vi "PSLDAQ_Close.vi"(0 "Handle In":T1) -> ()   [LabVIEW 2010]
doc: "1. 설명\n a. 장치와 통신 연결 기능 비활성화 및 할당된 메모리 제거\n\n2. 기능\n a. PSLDAQ_Open 함수에서 할당된 메모리, 쓰레드 제거\n b. PSL-DAQ 장치와 통신 연결 비활성화, 모든 기능 중지\n \n3. 터미널\n a. 터미널 입력\n ○ Handle In : 장치 핸들\n\n4. 주의\n a. PSLDAQ_Open 함수를 사용한 경우 반드시 PSLDAQ_Close 함수를 사용해야 함. \n b. 모든 함수를 사용한 후 호출함.\n c. PSLDAQ_Close 함수 사용 후 다시 PSLDAQ_Open 함수 사용 가능"
uses:
  PSLDAQ_Dll.dll
panel:
  # "PSLDAQ_Close\n\n1. 설명\n  a. 장치와 통신 연결 기능 비활성화 및 할당된 메모리 제거\n\n2. 기능\n  a. PSLDAQ_Open 함수에서 할당된 메모리, 쓰레드 제거\n  b. PSL-DAQ 장치와 통신 연결 비활성화, 모든 기능 중지\n        \n3. 터미널\n  a. 터미널 입력\n    ○ Handle In : 장치 핸들\n\n4. 주의\n  a. PSLDAQ_Open 함수를 사용한 경우 반드시 PSLDAQ_Close 함수를 사용해야 함.  \n  b. 모든 함수를 사용한 후 호출함.\n  c. PSLDAQ_Close 함수 사용 후 다시 PSLDAQ_Open 함수 사용 가능"
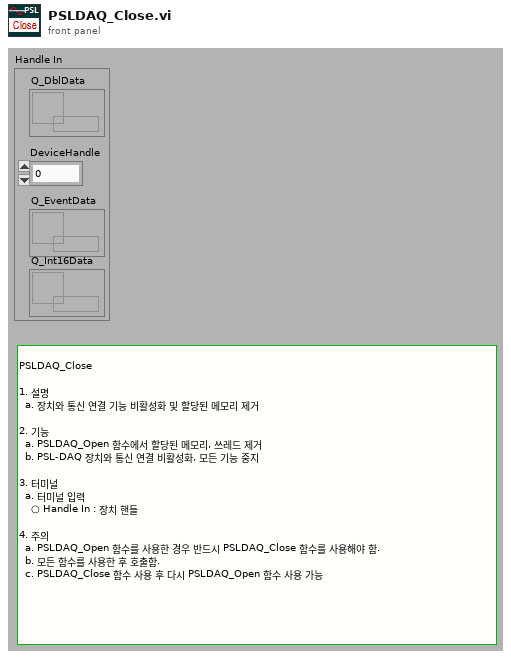
[diagram p1: front panel]
types:
  T1 = cluster{"Q_DblData":refnum<queue>, "DeviceHandle":u32, "Q_EventData":refnum<queue>, "Q_Int16Data":refnum<queue>}
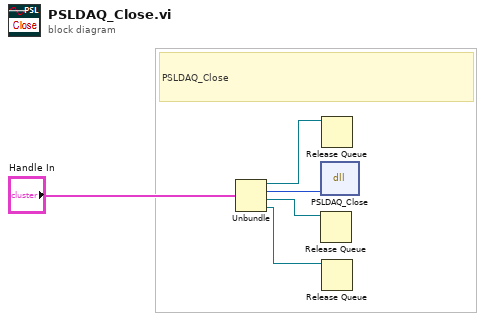
[diagram p0: block diagram]
diagram:
  # "PSLDAQ_Close"
  n1 = Unbundle("Handle In") -> ("Q_DblData"=w3:refnum<queue>, "DeviceHandle"=w5:u32, "Q_EventData"=w4:refnum<queue>, "Q_Int16Data"=w1:refnum<queue>)
  n2 = dll-call lib="D:/PSL-DAQ LabVIEW Library/PSLDAQ_Dll.dll" fn="PSLDAQ_Close"("DeviceHandle"=w5) -> ()  [unwired: 5 in, 2 out]
  n3 = Release Queue(queue=w4) -> ()  [unwired: 2 in, 3 out]
  n4 = Release Queue(queue=w3) -> ()  [unwired: 2 in, 3 out]
  n5 = Release Queue(queue=w1) -> ()  [unwired: 2 in, 3 out]
